vi "FPGA_RS232DigitalReader.vi"   [LabVIEW 2014]
uses:
  <vilib>/platform/TimedLoop/XDataNode/XDataNode.xnode
  <vilib>/Platform/TimedLoop/XDataNode/nitl_modes.ctl
  <vilib>/Platform/TimedLoop/XDataNode/XDNodeRunTimeDep.lvlib
  <vilib>/Platform/TimedLoop/XDataNode/wakeup.ctl
  <vilib>/Platform/TimedLoop/XDataNode/timing_clust.ctl
  <vilib>/eio/EIONode/EIONode.xnode
  <vilib>/rvi/eio/common/nirviEmuTemplateMethod_errors.vi
types:
  T1 = typedef "XDNodeRunTimeDep.lvlib/timing_clust.ctl" = cluster{"Expected End [f-1]":u64, "Actual End [f-1]":u64, "Finished Late? [f-1]":bool, "Expected End [i-1]":u64, "Actual End [i-1]":u64, "Finished Late? [i-1]":bool, "Expected Start [i]":u64, "Actual Start [i]":u64, "Expected Start [f]":u64, "Actual Start [f]":u64, "Source Name":string, "Structure Name":string, "Period":i64, "Deadline":i64, "Offset":i64, "Start":i64, "Priority":i32, "Timeout":i32, "Mode":T2, "Wakeup Reason":T3, "Error":errorcluster, "Source Type":string, "Secondary Source Type":string, "Global End Time":u64, "Global Start Time":u64, "Frame Duration":u64, "Iteration Duration":u64, "Assigned CPU":i32, "I/O Scan Engine Mode":u32}
  T2 = typedef "XDNodeRunTimeDep.lvlib/nitl_modes.ctl" = enum32{"No Change", "Process missed periods, maintain original phase", "Discard missed periods, maintain original phase", "Process missed periods, ignore original phase", "Discard missed periods, ignore original phase"}
  T3 = typedef "XDNodeRunTimeDep.lvlib/wakeup.ctl" = enum32{"Normal", "Aborted", "Asynchronous wakeup", "Timing source error", "Timed loop error", "Timeout"}
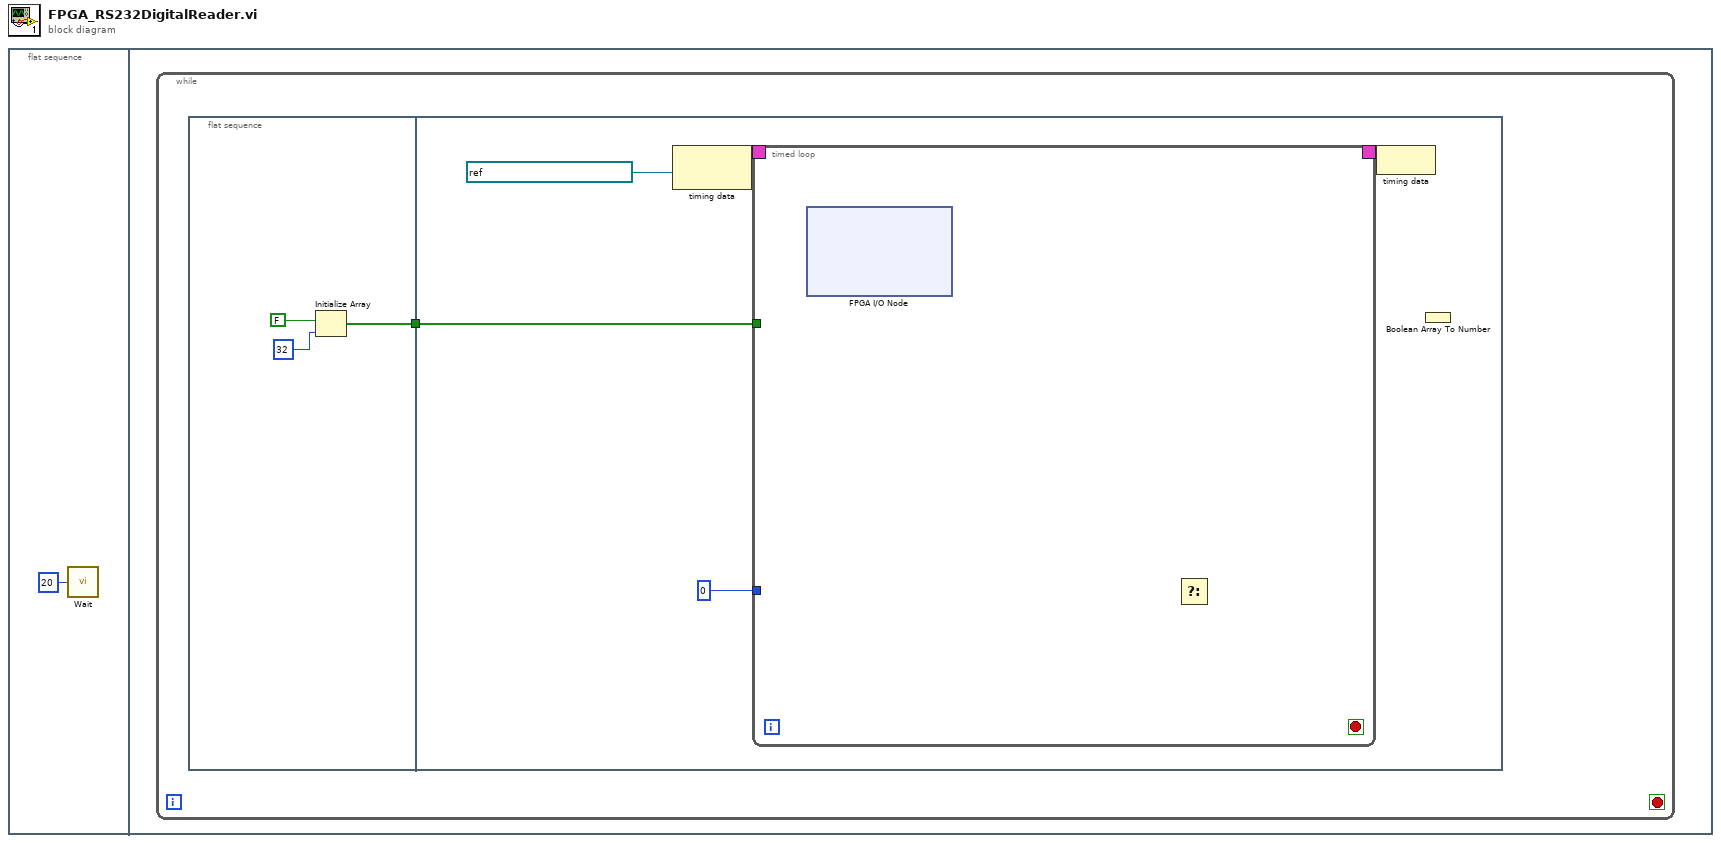
[diagram p0: block diagram]
diagram:
  n1 = flat-sequence {
    frame #0 {
      n2 = call "Wait"("Count(mSec)"=u32 20) -> ()  [unwired: 1 out]
    }
    frame #1 {
      n3 = while {
        stop <- _ stop-if-true
        n4 = flat-sequence {
          tunnel: [w3] -> w2
          tunnel: w2 -> [w7]
          frame #0 {
            n5 = Initialize Array(FALSE, 32 ("dimension size")) -> (w3:bool[])
          }
          frame #1 {
            n6 = node-c288(refnum<k21> "40 MHz Onboard Clock" ("Source Name")) -> (w10:T1)
            n7 = timed-loop {
              timing: w10 -> [_]
              timing-out: [_] -> w9
              tunnel: w7 -> [_]
              tunnel: i16 0 -> [_]
              stop <- _ stop-if-true
              n8 = xnode "FPGA I/O Node"() -> ()  [unwired: 4 in, 8 out]
              n9 = Select() -> ()  [unwired: 3 in, 1 out]
            }
            n10 = node-c288(w9) -> ()
            n11 = Boolean Array To Number() -> ()  [unwired: 1 in, 1 out]
          }
        }
      }
    }
  }
